vi "Create Manager.Text.INI.vi"(4 "write delay (ms)":i32, 5 "ConfigManager.Text.INI":refnum<class "ConfigManager.Text.INI.lvclass">, 6 "read-only?":bool, 8 "error in (no error)":errorcluster, 9 "Create if Non Existent? (T)":bool=TRUE, 11 "filepath":path) -> (0 "error out":errorcluster, 2 "CfgManager.Text Public Events":T1, 3 "ConfigManager.Text.INI out":refnum<class "ConfigManager.Text.INI.lvclass">)   [LabVIEW 2013, in "CfgManager.Text.lvlib" / "ConfigManager.Text.INI.lvclass"]
uses:
  ConfigManager.Text.INI.lvclass
  Manager.Text/PublicEvents -- Cluster.ctl
  Manager.Text/ConfigManager.Text.lvclass
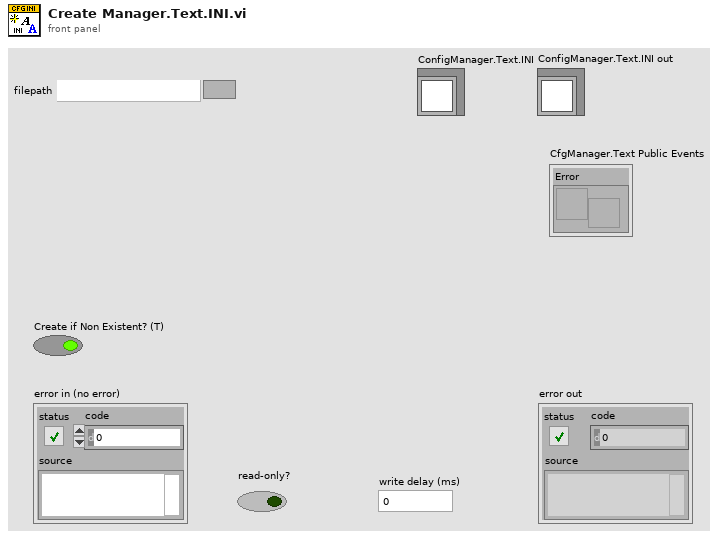
[diagram p1: front panel]
types:
  T1 = typedef "CfgManager.Text.lvlib/ConfigManager.Text.lvclass/PublicEvents -- Cluster.ctl" = cluster{"Error":refnum<user-event>}
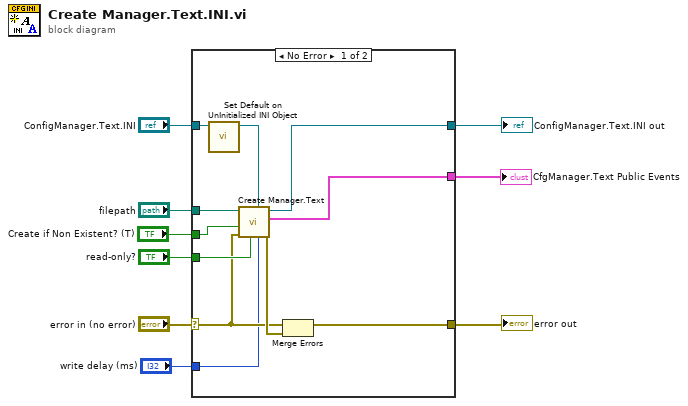
[diagram p0: block diagram]
diagram:
  n1 = case shown="No Error" "error in (no error)" {
    selector: "error in (no error)" -> [w17 w21]
    tunnel: "ConfigManager.Text.INI" -> [w13 w22]
    tunnel: [w16 w22] -> w3
    tunnel: "filepath" -> [w20 _]
    tunnel: [w14 w21] -> w6
    tunnel: "read-only?" -> [w19 _]
    tunnel: [w15 _] -> w4
    tunnel: "write delay (ms)" -> [w11 _]
    tunnel: "Create if Non Existent? (T)" -> [w10 _]
    frame No Error {
      n2 = call "Set Default on UnInitialized INI Object.vi"("ConfigManager.Text.INI"=w13) -> ("ConfigManager.Text.INI"=w12:refnum<class "ConfigManager.Text.INI.lvclass">)  [unwired: 10 in]
      n3 = call "Create Manager.Text.vi"("write delay (ms)"=w11, "ConfigManager.Text"=w12, "read-only?"=w19, "error in (no error)"=w17, "Create if Non Existent? (T)"=w10, "filepath"=w20) -> ("error out"=w18:errorcluster, "CfgManager.Text Public Events"=w15:T1, "ConfigManager.Text out"=w16:refnum<class "ConfigManager.Text.INI.lvclass">)  [unwired: 3 in]
      n4 = Merge Errors(w17, w18) -> (w14:errorcluster)
    }
    frame Error {
    }
  }
  "ConfigManager.Text.INI out" <- w3
  "error out" <- w6
  "CfgManager.Text Public Events" <- w4
